vi "Init_Subvi's.vi"(11 "error in (no error)":errorcluster) -> (4 "Init Reference":T1, 15 "error out":errorcluster)   [LabVIEW 2021]
uses:
  Controls/Init_TypeDef.ctl
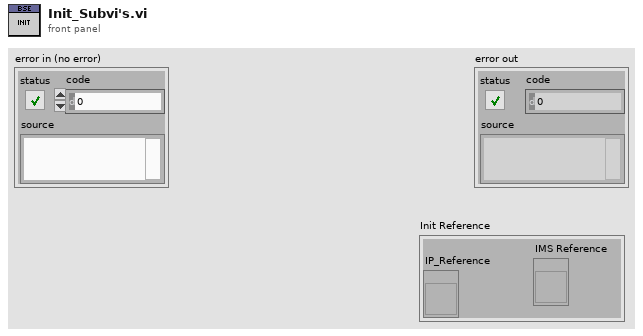
[diagram p1: front panel]
types:
  T1 = typedef "Init_TypeDef.ctl" = cluster{"IP_Reference":refnum<vi>, "IMS Reference":refnum<vi>}
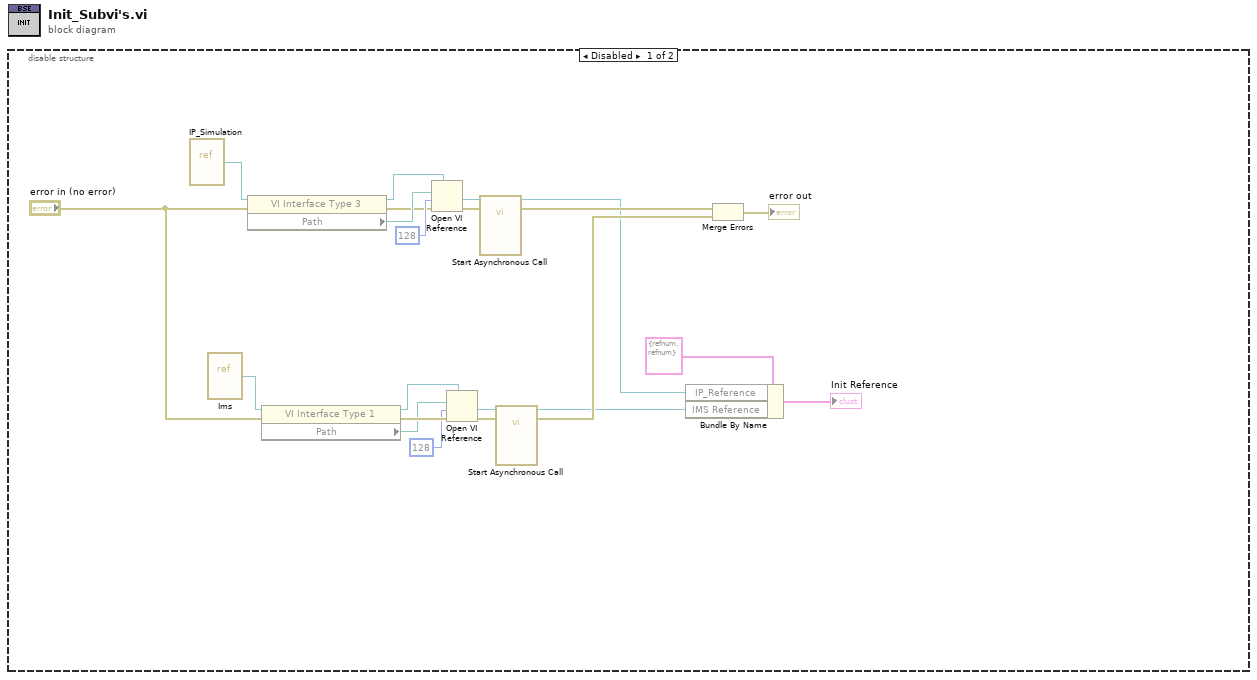
[diagram p0: block diagram]
diagram:
  n1 = disable-structure shown="Disabled" {
    frame Disabled {
      n2 = vi-ref "IP_Simulation.vi"() -> (w22:refnum<vi>)
      n3 = vi-ref "Ims.vi"() -> (w1:refnum<vi>)
      n4 = property class="VI Interface Type 3"(reference=w22, error in="error in (no error)") -> (reference out=w21:refnum<vi>, error out=w17:errorcluster, "Path"=w20:path)
      n5 = property class="VI Interface Type 1"(reference=w1, error in="error in (no error)") -> (reference out=w6:refnum<vi>, error out=w9:errorcluster, "Path"=w7:path)
      n6 = Open VI Reference(type specifier VI Refnum (for type only)=w21, vi path=w20, options=128, error in (no error)=w17) -> (vi reference=w18:refnum<vi>, error out=w16:errorcluster)  [unwired: 2 in]
      n7 = Open VI Reference(type specifier VI Refnum (for type only)=w6, vi path=w7, options=128, error in (no error)=w9) -> (vi reference=w3:refnum<vi>, error out=w10:errorcluster)  [unwired: 2 in]
      n8 = call-by-ref "Start Asynchronous Call"(reference=w18, error in=w16) -> (reference out=w11:refnum<vi>, error out=w14:errorcluster)  [unwired: 10 in, 2 out]
      n9 = call-by-ref "Start Asynchronous Call"(reference=w3, error in=w10) -> (reference out=w2:refnum<vi>, error out=w13:errorcluster)  [unwired: 8 in, 2 out]
      n10 = Bundle By Name(cluster=T1 {"IP_Reference"=refnum, "IMS Reference"=refnum} ("input cluster"), "IP_Reference"=w11, "IMS Reference"=w2) -> (→"Init Reference":T1)
      n11 = Merge Errors(w14, w13) -> (→"error out":errorcluster)
    }
    frame Enabled {
    }
  }
